vi "Test and Make Batch.vi"() -> ()   [LabVIEW 2010]
doc: "This program has two purposes. Firstly, it tests the functionality of \"MMB SubVI.vi\", which is a subVI implementation of \"MMB.vi\", the Moving Message Board VI. The user defines the parameters in the top section of the front panel. The parameter set can be tested to ensure proper operation via the \"Test\" button. When the \"Test\" button is clicked, it will pass the following inputs to the subVI: the path of the configuration file (a required input), a string with the message to be displayed (a required input), an integer with the delay time (a required input), an integer with the repeat or hold value (a required input), a cluster with the \"on\" color of the LED's in the display (a recommended input), a cluster with the \"off\" color of the LED's in the display (a recommended input), an enum with the operating mode (a required input), a cluster containing the LED width and height (a recommended input), and a cluster containing the display size width and height (based on number of LED's in the array, a recommended input).\n\nThe second purpose of this program is to build a batch file with each row being a set of parameters to be used via the \"Run Batch.vi\" and \"MMB SubVI.vi\" files. The user defines the parameters in the top section of the front panel. The parameter set can be tested to ensure proper operation via the \"Test\" button. When the parameters are correct, the \"Generate Line\" button will transfer them to the batch parameters array in the lower section of the front panel. The \"Delete Last Line\" button will remove the last line from the batch parameters array. The \"Clear All\" button will completely clear the array. The \"Load File\" button will load an existing batch parameters array and display it. The \"Write File\" button will write the batch parameters array to a file. The \"Stop\" button will end program execution."
uses:
  <vilib>/Utility/miscctls.llb/LVBoundsTypeDef.ctl
  <vilib>/Utility/file.llb/Read From Spreadsheet File (string).vi
  <vilib>/Utility/file.llb/Write To Spreadsheet File (string).vi
panel:
  in  "Default":bool
  in  "LED Off Color":u32(colorbox)
  in  "LED On Color":u32(colorbox)=6291200
  in  "Test":bool
  in  "Load":bool
  in  "Clear All":bool
  in  "Del Last":bool
  in  "Write":bool
  in  "stop":bool
  in  "Line":bool
  in  "Array":string[][](array[string])
  in  "Mode":T1(ring)
  in  "Repeat/Hold":u64=1 min=1 step=1
  in  "Display Size":T2={"Width"=60, "Height"=17} {"Width" min=1 step=1; "Height" min=1 step=1}
  in  "LED Size":T2={"Width"=17, "Height"=17} {"Width" min=1 step=1; "Height" min=1 step=1}
  in  "Delay":u32(knob)=50 step=1 scale=0.0..10000.0
  in  "Message":string="Hello"
  in  "Config Path":path=path "c:/Ed's Files/LabVIEW Files/My Code/Moving Message Board/mmb.ini" caption="Configuration File Path"
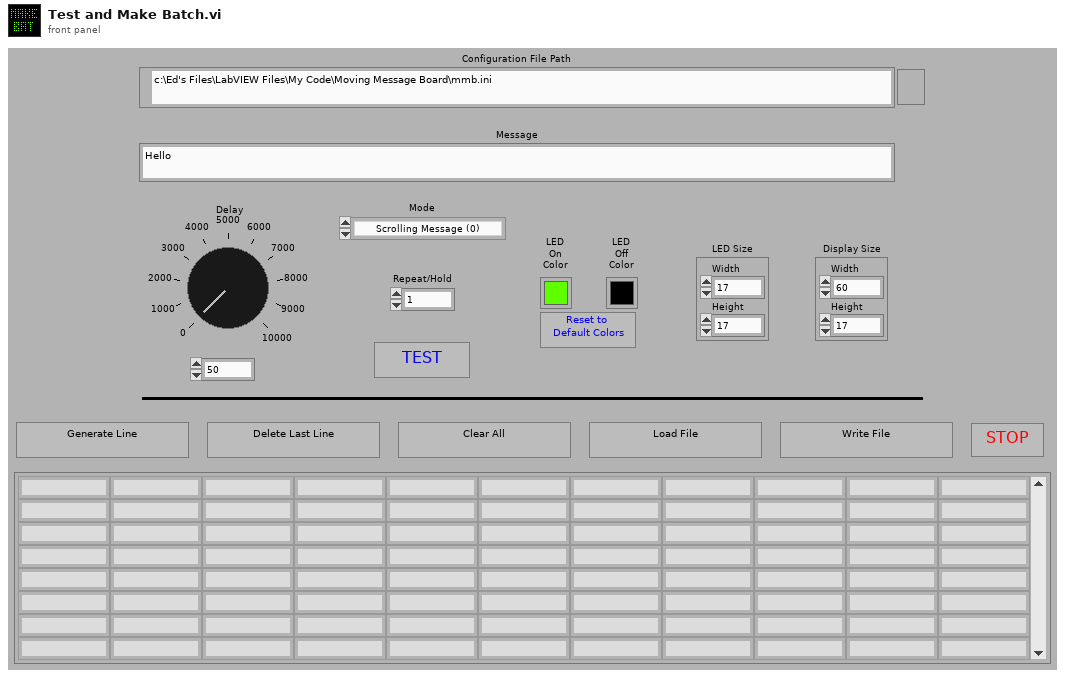
[diagram p1: front panel]
types:
  T1 = enum16{"Scrolling Message (0)", "Non-Scrolling Message (1)", "Fade In (2)", "Fade Out (3)", "Blink (4)", "Fly Up (5)", "Fall Down (6)", "Dissolve In (7)", "Dissolve Out (8)", "Random Pattern (9)"}
  T2 = typedef "LVBoundsTypeDef.ctl" = cluster{"Width":u32, "Height":u32}
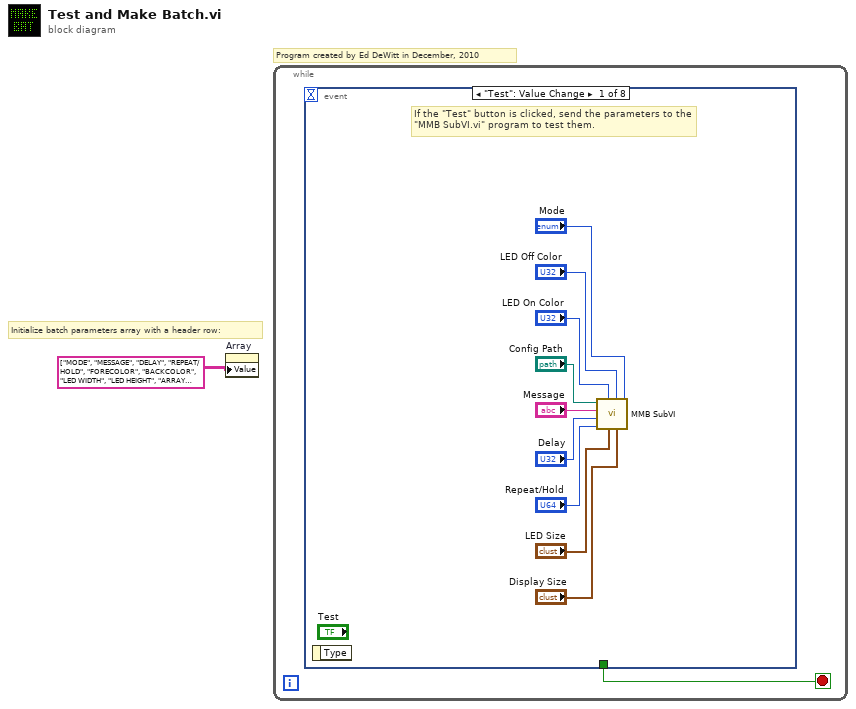
[diagram p0: block diagram]
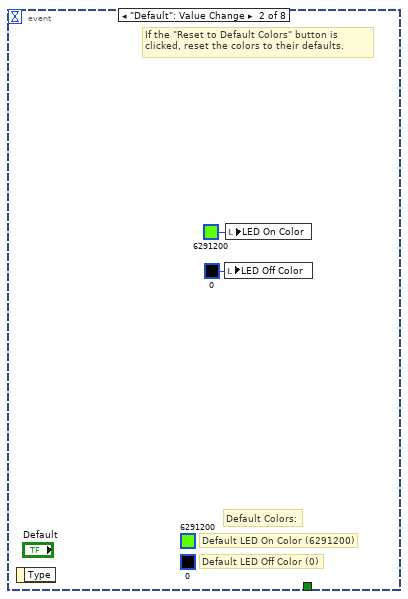
[diagram p2: hidden frame]
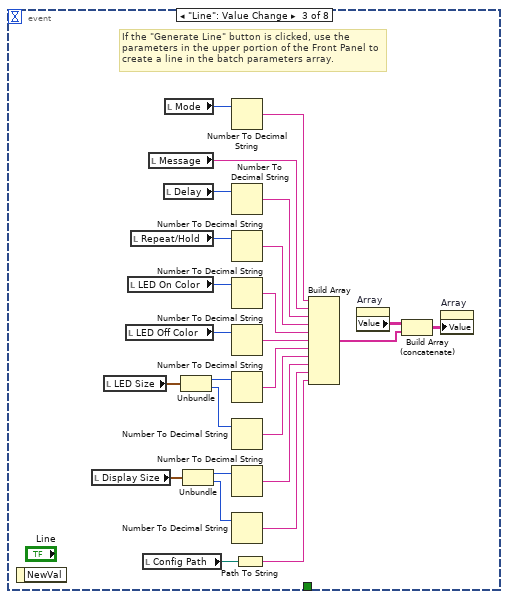
[diagram p3: hidden frame]
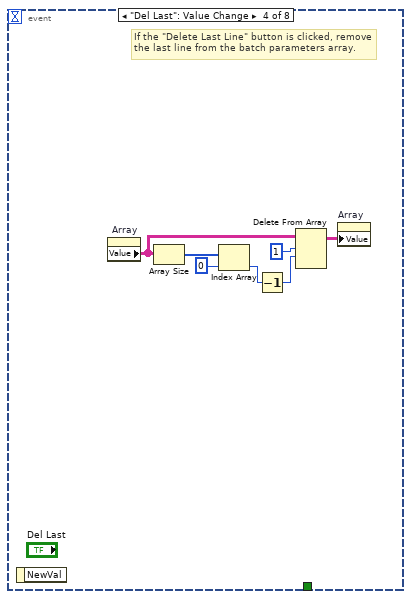
[diagram p4: hidden frame]
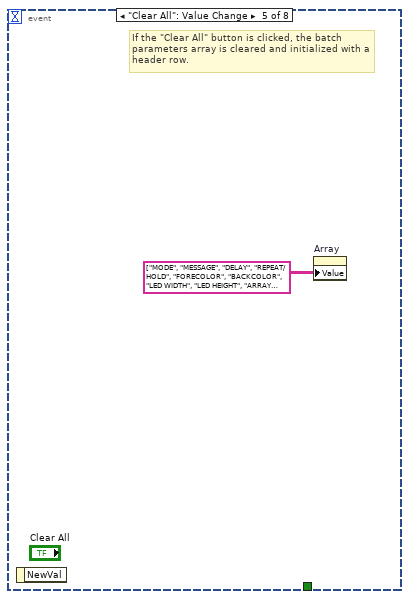
[diagram p5: hidden frame]
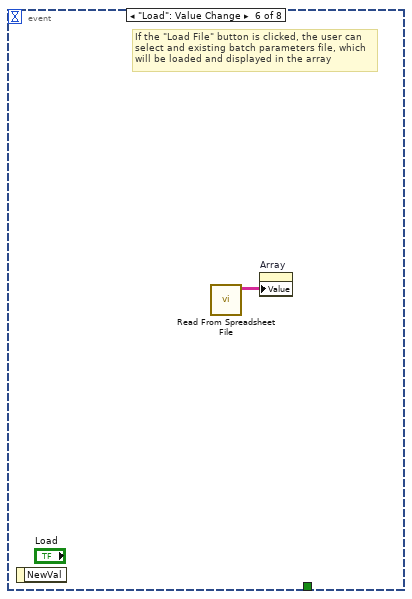
[diagram p6: hidden frame]
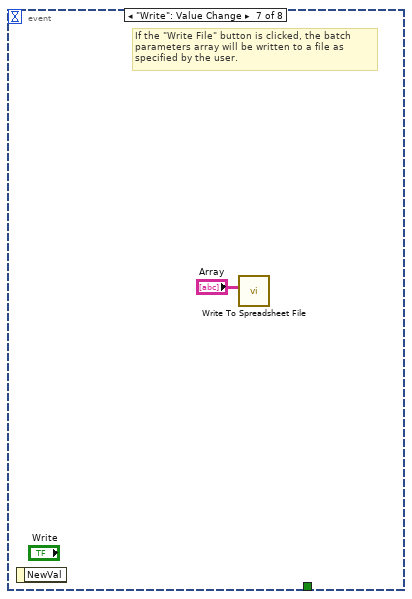
[diagram p7: hidden frame]
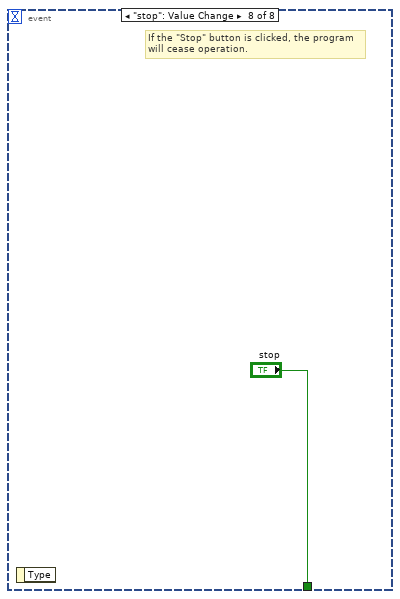
[diagram p8: hidden frame]
diagram:
  # "Initialize batch parameters array with a header row:"
  # "Program created by Ed DeWitt in December, 2010"
  n1 = property on="Array" class="Arr (strict)"("Value"=string[][] [["MODE", "MESSAGE", "DELAY", "REPEAT/HOLD", "FORECOLOR", "BACKCOLOR", "LED WIDTH", "LED HEIGHT", "ARRAY WIDTH", "ARRAY HEIGHT", "CONFIG FILE PATH"]]) -> ()  [unwired: 2 in, 2 out]
  n2 = while {
    stop <- w2 stop-if-true
    n3 = event shown="[0] \"Test\": Value Change" {
      selector: _ -> [_ _ _ _ _ _ _ _]
      dyn-events: _ -> [_ _ _ _ _ _ _ _]
      timeout: _ -> [_ _ _ _ _ _ _ _]
      tunnel: [_ _ _ _ _ _ _ "stop"] -> w2
      event "Test": Value Change {
        # "If the \"Test\" button is clicked, send the parameters to the \"MMB SubVI.vi\" program to test them."
        n4 = event-data() -> ()  [unwired: 1 in, 1 out]
        n5 = call "MMB SubVI.vi"("Mode"="Mode", "Array Size"="Display Size", "LED Off Color"="LED Off Color", "LED Size"="LED Size", "LED On Color"="LED On Color", "Repeat/Hold"="Repeat/Hold", "Delay"="Delay", "Message"="Message", "Config Path"="Config Path") -> ()  [unwired: 3 in]
      }
      event "Default": Value Change {
        (unwired) u32 0 ("BackColor")
        (unwired) u32 6291200 ("ForeColor")
        # "Default Colors:"
        # "Default LED On Color (6291200)"
        # "Default LED Off Color (0)"
        # "If the \"Reset to Default Colors\" button is clicked, reset the colors to their defaults."
        n6 = event-data() -> ()  [unwired: 1 in, 1 out]
        n7 = local write "LED Off Color"(u32 0 ("BackColor")) -> ()
        n8 = local write "LED On Color"(u32 6291200 ("ForeColor")) -> ()
      }
      event "Line": Value Change {
        # "If the \"Generate Line\" button is clicked, use the parameters in the upper portion of the Front Panel to create a line in the batch parameters array."
        n9 = event-data() -> ()  [unwired: 1 in, 1 out]
        n10 = local read "Display Size"() -> (w15:T2)
        n11 = local read "LED Size"() -> (w16:T2)
        n12 = local read "LED Off Color"() -> (w17:u32)
        n13 = local read "LED On Color"() -> (w18:u32)
        n14 = local read "Repeat/Hold"() -> (w19:u64)
        n15 = local read "Config Path"() -> (w14:path)
        n16 = local read "Message"() -> (w21:string)
        n17 = local read "Delay"() -> (w20:u32)
        n18 = local read "Mode"() -> (w22:T1)
        n19 = Unbundle(w16) -> ("Width"=w34:u32, "Height"=w32:u32)
        n20 = Unbundle(w15) -> ("Width"=w30:u32, "Height"=w28:u32)
        n21 = Number To Decimal String(number=w22) -> (decimal integer string=w39:string)  [unwired: 1 in]
        n22 = Number To Decimal String(number=w20) -> (decimal integer string=w38:string)  [unwired: 1 in]
        n23 = Number To Decimal String(number=w19) -> (decimal integer string=w37:string)  [unwired: 1 in]
        n24 = Number To Decimal String(number=w18) -> (decimal integer string=w36:string)  [unwired: 1 in]
        n25 = Number To Decimal String(number=w17) -> (decimal integer string=w35:string)  [unwired: 1 in]
        n26 = Number To Decimal String(number=w34) -> (decimal integer string=w33:string)  [unwired: 1 in]
        n27 = Number To Decimal String(number=w32) -> (decimal integer string=w31:string)  [unwired: 1 in]
        n28 = Number To Decimal String(number=w30) -> (decimal integer string=w29:string)  [unwired: 1 in]
        n29 = Number To Decimal String(number=w28) -> (decimal integer string=w27:string)  [unwired: 1 in]
        n30 = Path To String(path=w14) -> (string=w26:string)
        n31 = Build Array(w39, w21, w38, w37, w36, w35, w33, w31, w29, w27, w26) -> (w25:string[])
        n32 = property on="Array" class="Arr (strict)"() -> ("Value"=w24:string[][])  [unwired: 2 in, 2 out]
        n33 = Build Array (concatenate)(w24, w25) -> (w23:string[][])
        n34 = property on="Array" class="Arr (strict)"("Value"=w23) -> ()  [unwired: 2 in, 2 out]
      }
      event "Del Last": Value Change {
        # "If the \"Delete Last Line\" button is clicked, remove the last line from the batch parameters array."
        n35 = event-data() -> ()  [unwired: 1 in, 1 out]
        n36 = property on="Array" class="Arr (strict)"() -> ("Value"=w44:string[][])  [unwired: 2 in, 2 out]
        n37 = Array Size(array=w44) -> (size(s)=w46:i32[])
        n38 = Index Array(array=w46, index=0) -> (element=w41:i32)
        n39 = Decrement(x=w41) -> (x-1=w40:i32)
        n40 = Delete From Array(array=w44, length=1, index (row)=w40) -> (array with subset deleted=w42:string[][])  [unwired: 1 in, 1 out]
        n41 = property on="Array" class="Arr (strict)"("Value"=w42) -> ()  [unwired: 2 in, 2 out]
      }
      event "Clear All": Value Change {
        # "If the \"Clear All\" button is clicked, the batch parameters array is cleared and initialized with a header row."
        n42 = event-data() -> ()  [unwired: 1 in, 1 out]
        n43 = property on="Array" class="Arr (strict)"("Value"=string[][] [["MODE", "MESSAGE", "DELAY", "REPEAT/HOLD", "FORECOLOR", "BACKCOLOR", "LED WIDTH", "LED HEIGHT", "ARRAY WIDTH", "ARRAY HEIGHT", "CONFIG FILE PATH"]]) -> ()  [unwired: 2 in, 2 out]
      }
      event "Load": Value Change {
        # "If the \"Load File\" button is clicked, the user can select and existing batch parameters file, which will be loaded and displayed in the array"
        n44 = event-data() -> ()  [unwired: 1 in, 1 out]
        n45 = call-poly <vilib>:"Read From Spreadsheet File.vi"() -> ("all rows"=w48:string[][])  [unwired: 7 in, 4 out]
        n46 = property on="Array" class="Arr (strict)"("Value"=w48) -> ()  [unwired: 2 in, 2 out]
      }
      event "Write": Value Change {
        # "If the \"Write File\" button is clicked, the batch parameters array will be written to a file as specified by the user."
        n47 = event-data() -> ()  [unwired: 1 in, 1 out]
        n48 = call-poly <vilib>:"Write To Spreadsheet File.vi"("2D data"="Array") -> ()  [unwired: 7 in, 1 out]
      }
      event "stop": Value Change {
        # "If the \"Stop\" button is clicked, the program will cease operation."
        n49 = event-data() -> ()  [unwired: 1 in, 1 out]
      }
    }
  }
